vi "setToSortBy.vi"(8 "error in (no error)":errorcluster, 10 "ToSortBy":dbl, 11 "BasicSortedNode in":refnum<class "BasicSortedNode.lvclass">) -> (0 "error out":errorcluster, 3 "BasicSortedNode out":refnum<class "BasicSortedNode.lvclass">)   [LabVIEW 2009, in "BasicSortedNode.lvclass"]
doc: "Sets the value of what is used to sort the list by."
uses:
  BasicSortedNode.lvclass
  BasicSortedNode.lvclass/BasicSortedNode.ctl
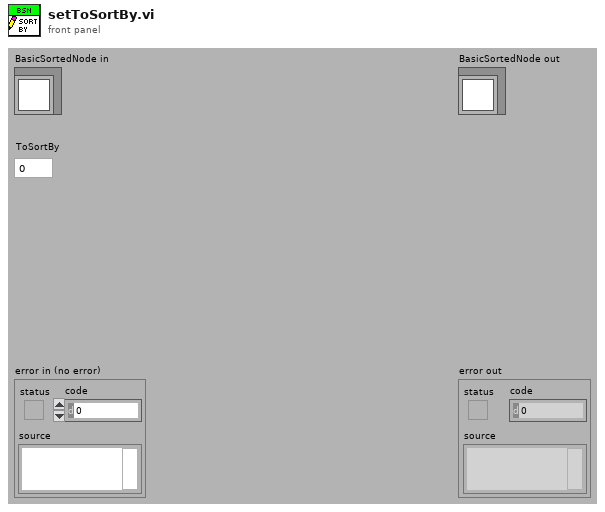
[diagram p1: front panel]
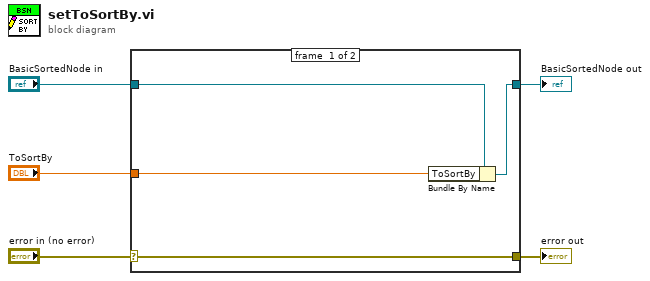
[diagram p0: block diagram]
diagram:
  n1 = case shown="No Error" "error in (no error)" {
    selector: "error in (no error)" -> [w9 w10]
    tunnel: [w9 w10] -> w4
    tunnel: [w7 w11] -> w2
    tunnel: "BasicSortedNode in" -> [w8 w11]
    tunnel: "ToSortBy" -> [w6 _]
    frame #0 {
      n2 = Bundle By Name(cluster=w8, "ToSortBy"=w6) -> (w7:refnum<class "BasicSortedNode.lvclass">)
    }
    frame #1 {
    }
  }
  "error out" <- w4
  "BasicSortedNode out" <- w2
